vi "close.vi"(8 "error in (no error)":errorcluster, 11 "controller in":refnum<class "controller.lvclass">) -> (0 "error out":errorcluster, 3 "controller out":refnum<class "controller.lvclass">)   [LabVIEW 2025, in "controller.lvclass"]
uses:
  controller.lvclass
  controller.lvclass/controller.ctl
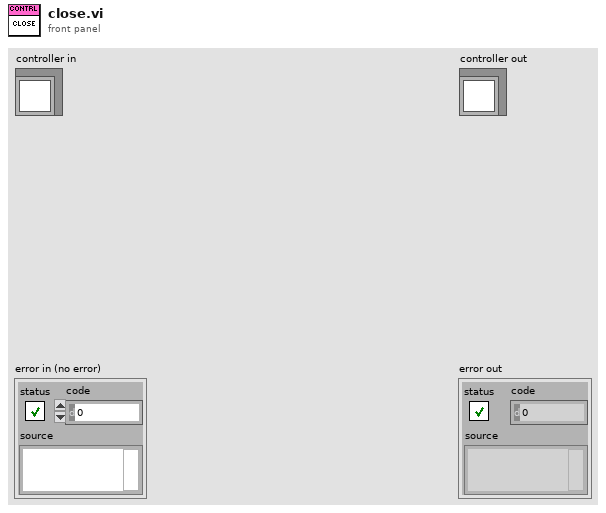
[diagram p1: front panel]
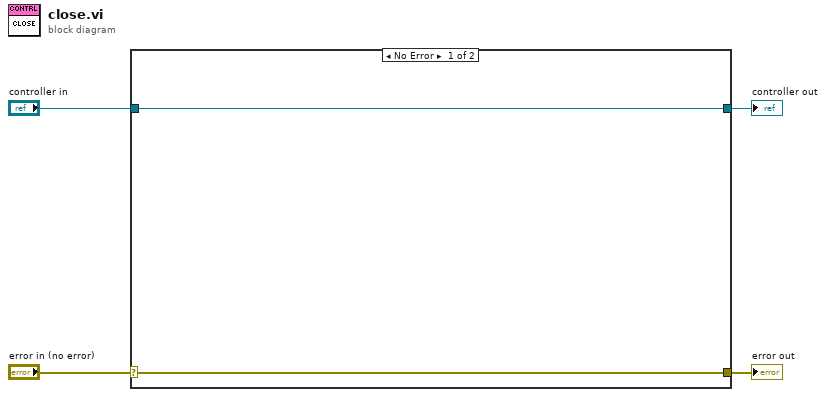
[diagram p0: block diagram]
diagram:
  n1 = case shown="No Error" "error in (no error)" {
    selector: "error in (no error)" -> [w5 w8]
    tunnel: [w5 w8] -> w3
    tunnel: [w6 w7] -> w1
    tunnel: "controller in" -> [w6 w7]
    frame No Error {
    }
    frame Error {
    }
  }
  "error out" <- w3
  "controller out" <- w1
